vi "Main.vi"   [LabVIEW 2019]
doc: "The myRIO Project template acquires acceleration data from the onboard accelerometer and displays the changes of acceleration values in a waveform chart."
uses:
  KNRm_ReMi_OS6_64Motor.lvlibp/KNRm_ReMi_Toolkit/IO/LowLevel/IO_Channel_RC.ctl
  KNRm_ReMi_OS6_64Motor.lvlibp
types:
  T1 = typedef "Image Type" = u32
  T2 = typedef "IMAQ Image.ctl" = refnum<image>
  T3 = typedef "KNRm_ReMi_OS6_64Motor.lvlibp/IO_Channel_RC.ctl" = enum16{"RC1", "RC2", "S1(EXTIOB)", "S2(EXTIOB)", "S3(EXTIOB)", "S4(EXTIOB)", "S5(EXTIOB)", "S6(EXTIOB)"}
  T4 = enum16{"UP IR1", "UP IR2", "Turn IR1 IR2", "UPL IR1 IR2 US1", "UPR IR1 IR2 US2"}
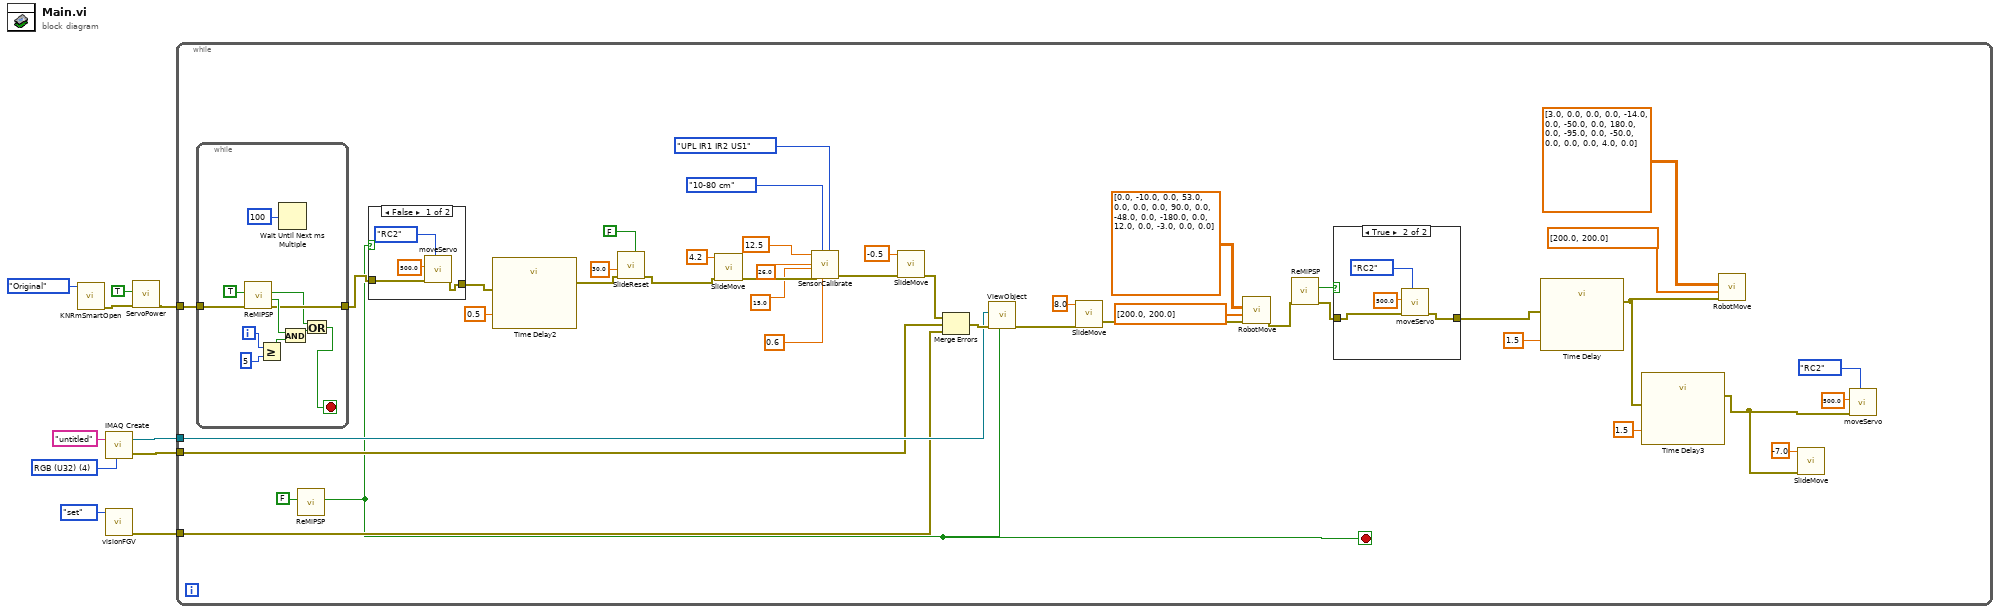
[diagram p0: block diagram]
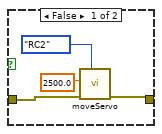
[diagram p2: hidden frame]
diagram:
  w5 = T1 4 items=["Grayscale (U8)", "Grayscale (I16)", "Grayscale (SGL)", "Complex (CSG)", "RGB (U32)", "HSL (U32)", "RGB (U64)", "Grayscale (U16)"] ("Image Type")
  n1 = call "KNRmSmartOpen.vi"("INI FPGA MODE"=enum16{"Original", "M4EXTIOB"}."Original") -> ("error out"=w10:errorcluster)  [unwired: 7 in, 3 out]
  n2 = call "IMAQ Create"("Image Name"="untitled", "Image Type"=w5) -> ("New Image"=w3:T2, "error out"=w2:errorcluster)  [unwired: 3 in]
  n3 = call "visionFGV.vi"("Function"=enum16{"set", "read", "close"}."set") -> ("error out"=w1:errorcluster)  [unwired: 9 in, 1 out]
  n4 = call "ServoPower.vi"("error in (no error)"=w10, "ServoENA"=TRUE) -> ("error out"=w7:errorcluster)  [unwired: 9 in]
  n5 = while {
    tunnel: w7 -> [w25]
    tunnel: w3 -> [w20]
    tunnel: w2 -> [w19]
    tunnel: w1 -> [w18]
    stop <- w16 stop-if-true
    n6 = while {
      tunnel: w25 -> [w77]
      tunnel: [w71] -> w17
      i -> [w75]
      stop <- w68 stop-if-true
      n7 = call "ReMiPSP.vi"("error in"=w77, "Green (T) /Yellow (F)"=TRUE) -> ("error out"=w71:errorcluster, "UserBtn"=w73:bool, "EMS"=w69:bool)  [unwired: 7 in]
      n8 = Greater Or Equal?(x=w75, y=5) -> (x >= y?=w72:bool)
      n9 = Wait Until Next ms Multiple(millisecond multiple=u32 100) -> ()  [unwired: 1 out]
      n10 = And(x=w73, y=w72) -> (x .and. y?=w70:bool)
      n11 = Or(x=w69, y=w70) -> (x .or. y?=w68:bool)
    }
    n12 = call "ReMiPSP.vi"("Green (T) /Yellow (F)"=FALSE) -> ("EMS"=w16:bool)  [unwired: 8 in, 2 out]
    n13 = case shown="False" w16 {
      tunnel: [w62 w66] -> w29
      tunnel: w17 -> [w63 w66]
      frame False {
        n14 = call "moveServo.vi"("Channel"=IO_Channel_RC."RC2", "error in (no error)"=w63, "Servo Position (us)"=500.0) -> ("error out"=w62:errorcluster)  [unwired: 8 in]
      }
      frame True {
      }
    }
    n15 = call "Time Delay2"("error in (no error)"=w29, "Delay Time (s)"=0.5) -> ("error out"=w28:errorcluster)  [unwired: 9 in]
    n16 = call "SlideReset.vi"("reverse LimBtn(F)"=FALSE, "error out"=w28, "speed"=30.0) -> ("error out 2"=w52:errorcluster)  [unwired: 8 in]
    n17 = call "SlideMove.vi"("error in"=w52, "SetCm"=4.2) -> ("error out"=w49:errorcluster)  [unwired: 9 in]
    n18 = call "SensorCalibrate.vi"("Set mode"=T4."UPL IR1 IR2 US1", "IR Err"=0.6, "type"=enum16{"10-80 cm", "4-30 cm"}."10-80 cm", "error in (no error)"=w49, "Speed"=15.0, "IR_Distance(CM)"=26.0, "USS_Distance(CM)"=12.5) -> ("error out"=w41:errorcluster)  [unwired: 4 in]
    n19 = call "SlideMove.vi"("error in"=w41, "SetCm"=-0.5) -> ("error out"=w40:errorcluster)  [unwired: 9 in]
    n20 = Merge Errors(w40, w19, w18) -> (w39:errorcluster)
    n21 = call "ViewObject.vi"("y"=w16, "error in"=w39, "New Image"=w20) -> ("error out"=w37:errorcluster)  [unwired: 6 in, 2 out]
    n22 = call "SlideMove.vi"("error in"=w37, "SetCm"=8.0) -> ("error out"=w34:errorcluster)  [unwired: 9 in]
    n23 = call "RobotMove.vi"("error in (no error)"=w34, "Speed ACC"=dbl[] [200.0, 200.0], "XYZ"=dbl[][] [[0.0, -10.0, 0.0], [53.0, 0.0, 0.0], [0.0, 90.0, 0.0], [-48.0, 0.0, -180.0], [0.0, 12.0, 0.0], [-3.0, 0.0, 0.0]]) -> ("error out"=w33:errorcluster)  [unwired: 5 in, 2 out]
    n24 = call "ReMiPSP.vi"("error in"=w33) -> ("error out"=w11:errorcluster, "EMS"=w12:bool)  [unwired: 8 in, 1 out]
    n25 = case shown="True" w12 {
      tunnel: w11 -> [w55 w59]
      tunnel: [w54 w58] -> w32
      frame False {
        n26 = call "moveServo.vi"("Channel"=IO_Channel_RC."RC2", "error in (no error)"=w55, "Servo Position (us)"=2500.0) -> ("error out"=w54:errorcluster)  [unwired: 8 in]
      }
      frame True {
        n27 = call "moveServo.vi"("Channel"=IO_Channel_RC."RC2", "error in (no error)"=w59, "Servo Position (us)"=500.0) -> ("error out"=w58:errorcluster)  [unwired: 8 in]
      }
    }
    n28 = call "Time Delay"("error in (no error)"=w32, "Delay Time (s)"=1.5) -> ("error out"=w23:errorcluster)  [unwired: 9 in]
    n29 = call "Time Delay3"("error in (no error)"=w23, "Delay Time (s)"=1.5) -> ("error out"=w21:errorcluster)  [unwired: 9 in]
    n30 = call "RobotMove.vi"("error in (no error)"=w23, "Speed ACC"=dbl[] [200.0, 200.0], "XYZ"=dbl[][] [[3.0, 0.0, 0.0], [0.0, -14.0, 0.0], [-50.0, 0.0, 180.0], [0.0, -95.0, 0.0], [-50.0, 0.0, 0.0], [0.0, 4.0, 0.0]]) -> ()  [unwired: 5 in, 3 out]
    n31 = call "SlideMove.vi"("error in"=w21, "SetCm"=-7.0) -> ()  [unwired: 9 in, 1 out]
    n32 = call "moveServo.vi"("Channel"=IO_Channel_RC."RC2", "error in (no error)"=w21, "Servo Position (us)"=500.0) -> ()  [unwired: 8 in, 1 out]
  }
